vi "chargetest.vi"(0 "stop":bool, 4 "Stop Time(s)":dbl, 5 "Stop Current(A)":dbl, 6 "Stop Capacity(Ah)":dbl, 7 "Stop Voltage(V)":dbl, 8 "Charge\\Discharge Current(A)":dbl, 9 "Charge\\Discharge Voltage(V)":dbl, 10 "Battery Mode":u8(ring) items=["Charge", "Discharge"], 11 "VISA resource name":refnum<visa-resource-name>) -> (1 "Read Voltage(V)":dbl format="%.2g", 2 "Read Current(A)":dbl format="%.2g")   [LabVIEW 2020]
uses:
  <instrlib>/IT-M3400/IT-M3400.lvlib
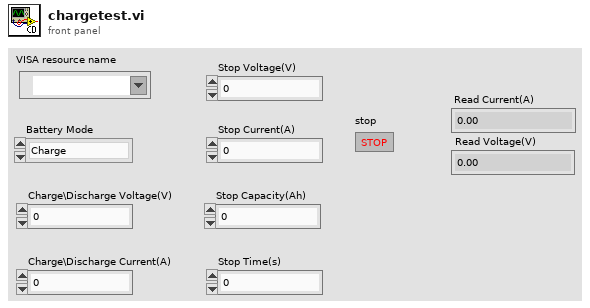
[diagram p1: front panel]
types:
  T1 = cluster{"Baud Rate":u32, "Parity":u16, "Data Bits":u16, "Stop Bits":u16, "Flow Control":u16}
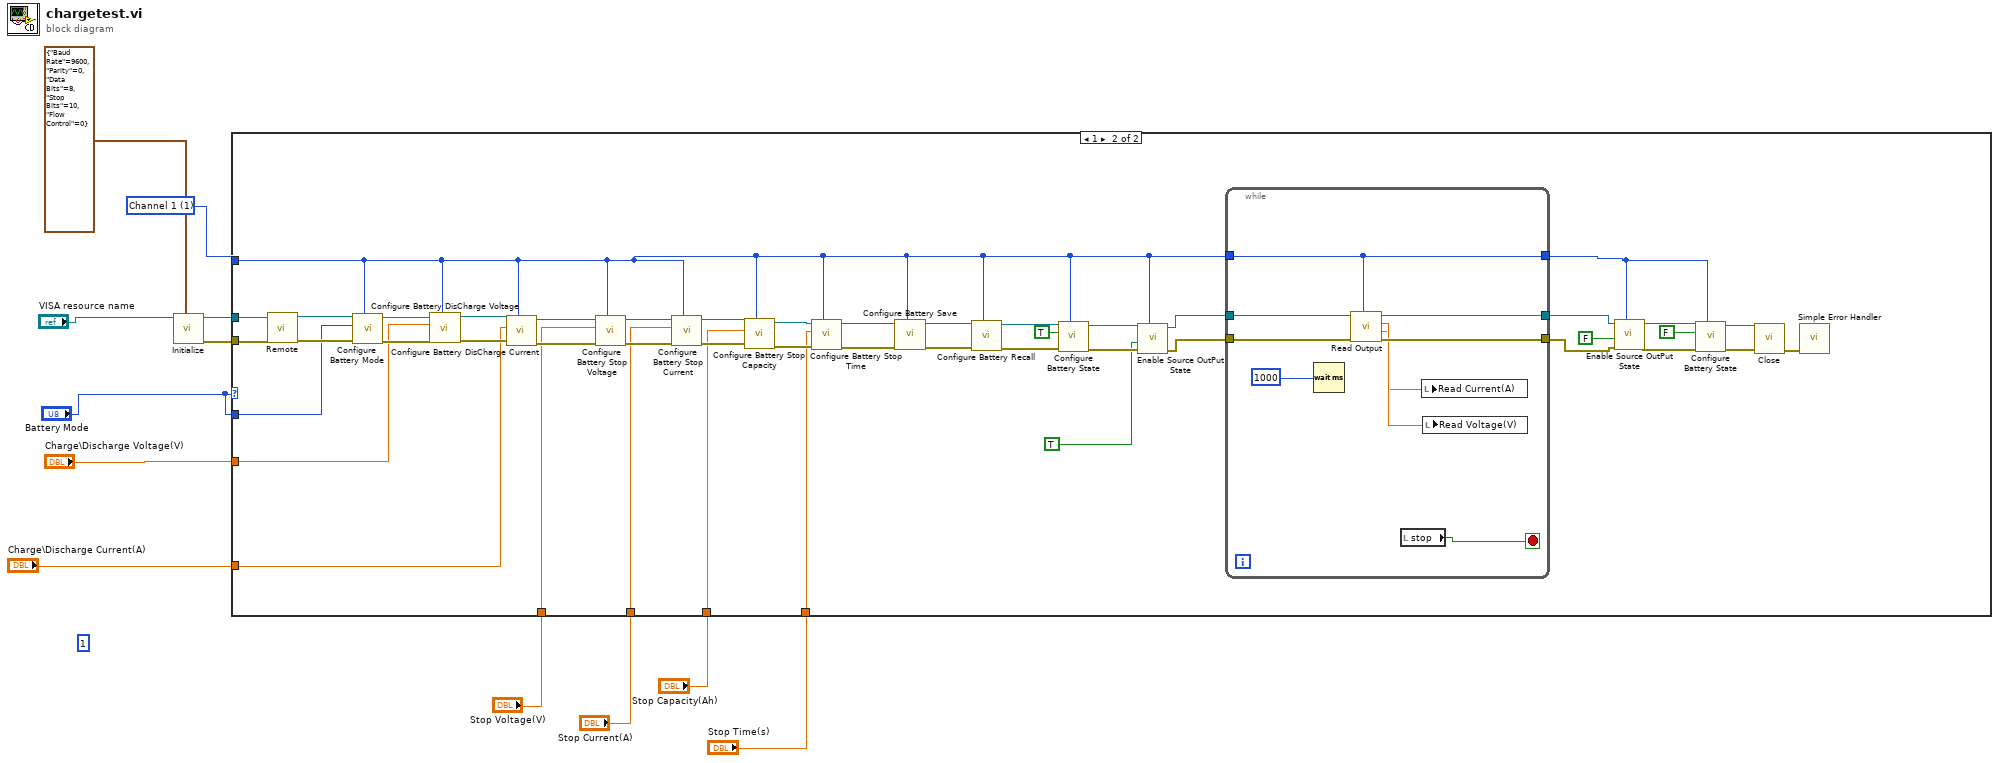
[diagram p0: block diagram]
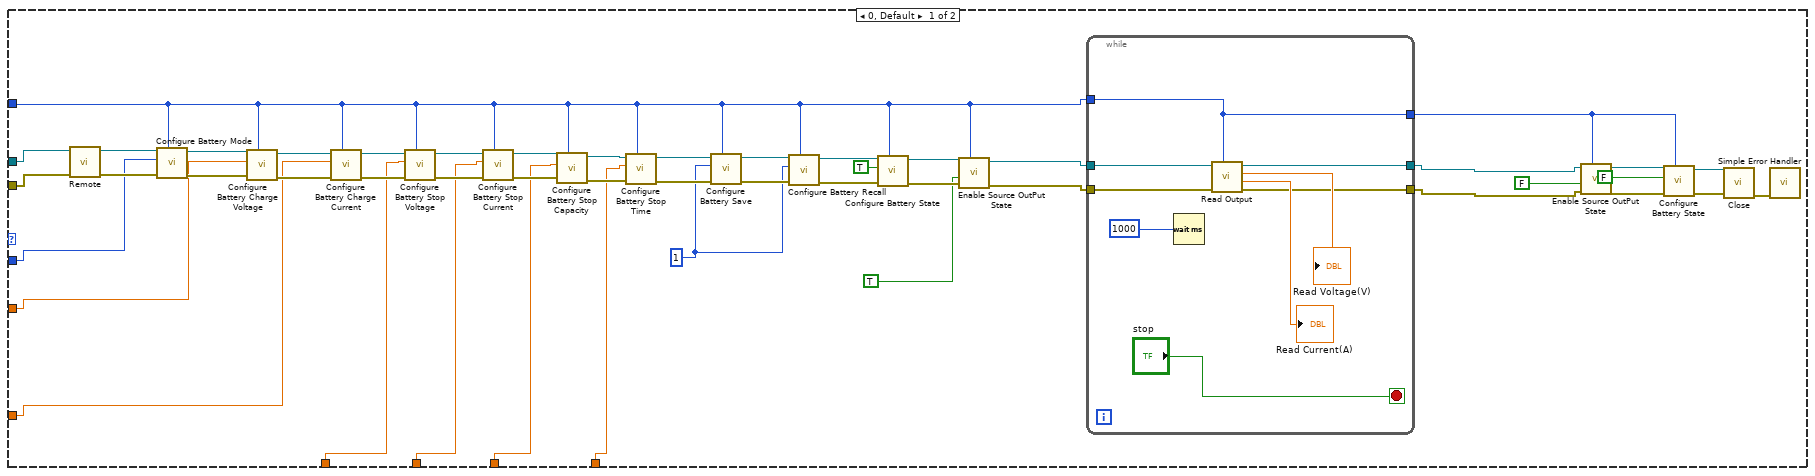
[diagram p2: hidden frame]
diagram:
  w2 = 1 items=["Channel 1"=1, "Channel 2"=2, "Channel 3"=3, "Channel 4"=4, "Channel 5"=5, "Channel 6"=6, "Channel 7"=7, "Channel 8"=8, "Channel 8"=9, "Channel 10"=10, "Channel 11"=11, "Channel 12"=12, "Channel 13"=13, "Channel 14"=14, "Channel 15"=15, "Channel 16"=16] ("Channel")
  (unwired) 1
  n1 = call <instrlib>:"Initialize.vi"("Serial Configuration"=T1 {"Baud Rate"=9600, "Parity"=0, "Data Bits"=8, "Stop Bits"=10, "Flow Control"=0}, "VISA resource name"="VISA resource name") -> ("error out"=w11:errorcluster, "VISA resource name out"=w12:refnum<visa-resource-name>)  [unwired: 8 in]
  n2 = case shown="1" "Battery Mode" {
    tunnel: "Battery Mode" -> [w26 w104]
    tunnel: w12 -> [w28 w103]
    tunnel: w11 -> [w27 w102]
    tunnel: "Charge\\Discharge Voltage(V)" -> [w25 w79]
    tunnel: "Charge\\Discharge Current(A)" -> [w24 w80]
    tunnel: "Stop Voltage(V)" -> [w23 w78]
    tunnel: "Stop Current(A)" -> [w22 w77]
    tunnel: "Stop Capacity(Ah)" -> [w21 w76]
    tunnel: "Stop Time(s)" -> [w20 w75]
    tunnel: w2 -> [w14 w72]
    frame 0, Default {
      w19 = u8 1 ("File")
      n3 = call <instrlib>:"Remote.vi"("error in"=w27, "VISA resource name"=w28) -> ("error out"=w58:errorcluster, "VISA resource name out"=w59:refnum<visa-resource-name>)  [unwired: 8 in]
      n4 = call <instrlib>:"Configure Battery Mode.vi"("Channel"=w14, "error in"=w58, "Battery Mode"=w26, "VISA resource name"=w59) -> ("error out"=w56:errorcluster, "VISA resource name out"=w57:refnum<visa-resource-name>)  [unwired: 6 in]
      n5 = call <instrlib>:"Configure Battery Charge Voltage.vi"("Channel"=w14, "error in"=w56, "Charge Voltage(V)"=w25, "VISA resource name"=w57) -> ("error out"=w54:errorcluster, "VISA resource name out"=w55:refnum<visa-resource-name>)  [unwired: 5 in]
      n6 = call <instrlib>:"Configure Battery Charge Current.vi"("Channel"=w14, "error in"=w54, "Charge Current(A)"=w24, "VISA resource name"=w55) -> ("error out"=w52:errorcluster, "VISA resource name out"=w53:refnum<visa-resource-name>)  [unwired: 6 in]
      n7 = call <instrlib>:"Configure Battery Stop Voltage.vi"("Channel"=w14, "error in"=w52, "Stop Voltage(V)"=w23, "VISA resource name"=w53) -> ("error out"=w50:errorcluster, "VISA resource name out"=w51:refnum<visa-resource-name>)  [unwired: 6 in]
      n8 = call <instrlib>:"Configure Battery Stop Current.vi"("Channel"=w14, "error in"=w50, "Stop Current(A)"=w22, "VISA resource name"=w51) -> ("error out"=w48:errorcluster, "VISA resource name out"=w49:refnum<visa-resource-name>)  [unwired: 6 in]
      n9 = call <instrlib>:"Configure Battery Stop Capacity.vi"("Channel"=w14, "error in"=w48, "Stop Capacity(Ah)"=w21, "VISA resource name"=w49) -> ("error out"=w46:errorcluster, "VISA resource name out"=w47:refnum<visa-resource-name>)  [unwired: 6 in]
      n10 = call <instrlib>:"Configure Battery Stop Time.vi"("Channel"=w14, "error in"=w46, "Stop Time(S)"=w20, "VISA resource name"=w47) -> ("error out"=w44:errorcluster, "VISA resource name out"=w45:refnum<visa-resource-name>)  [unwired: 6 in]
      n11 = call <instrlib>:"Configure Battery Save.vi"("Channel"=w14, "error in"=w44, "File"=w19, "VISA resource name"=w45) -> ("error out"=w42:errorcluster, "VISA resource name out"=w43:refnum<visa-resource-name>)  [unwired: 6 in]
      n12 = call <instrlib>:"Configure Battery Recall.vi"("Channel"=w14, "error in"=w42, "File"=w19, "VISA resource name"=w43) -> ("error out"=w40:errorcluster, "VISA resource name out"=w41:refnum<visa-resource-name>)  [unwired: 6 in]
      n13 = call <instrlib>:"Configure Battery State.vi"("Channel"=w14, "error in"=w40, "State"=TRUE, "VISA resource name"=w41) -> ("error out"=w38:errorcluster, "VISA resource name out"=w39:refnum<visa-resource-name>)  [unwired: 6 in]
      n14 = call <instrlib>:"Enable Source OutPut State.vi"("Channel"=w14, "error in"=w38, "State"=TRUE ("Enable Output|Intput"), "VISA resource name"=w39) -> ("error out"=w17:errorcluster, "VISA resource name out"=w18:refnum<visa-resource-name>)  [unwired: 6 in]
      n15 = while {
        tunnel: w18 -> [w66]
        tunnel: w17 -> [w65]
        tunnel: [w64] -> w16
        tunnel: [w63] -> w15
        tunnel: w14 -> [w60]
        tunnel: [w60] -> w13
        stop <- "stop" stop-if-true
        n16 = Wait (ms)(milliseconds to wait=1000) -> ()  [unwired: 1 out]
        n17 = call <instrlib>:"Read Output.vi"("Channel"=w60, "error in"=w65, "VISA resource name"=w66) -> ("error out"=w63:errorcluster, "Read Current(A)"=→"Read Current(A)":dbl, "Read Voltage(V)"=→"Read Voltage(V)":dbl, "VISA resource name out"=w64:refnum<visa-resource-name>)  [unwired: 5 in]
      }
      n18 = call <instrlib>:"Enable Source OutPut State.vi"("Channel"=w13, "error in"=w15, "State"=FALSE, "VISA resource name"=w16) -> ("error out"=w31:errorcluster, "VISA resource name out"=w34:refnum<visa-resource-name>)  [unwired: 6 in]
      n19 = call <instrlib>:"Configure Battery State.vi"("Channel"=w13, "error in"=w31, "State"=FALSE, "VISA resource name"=w34) -> ("error out"=w32:errorcluster, "VISA resource name out"=w33:refnum<visa-resource-name>)  [unwired: 6 in]
      n20 = call <instrlib>:"Close.vi"("error in"=w32, "VISA resource name"=w33) -> ("error out"=w36:errorcluster)  [unwired: 9 in]
      n21 = call <vilib>:"Simple Error Handler.vi"("error in (no error)"=w36) -> ()  [unwired: 4 in, 5 out]
    }
    frame 1 {
      n22 = call <instrlib>:"Remote.vi"("error in"=w102, "VISA resource name"=w103) -> ("error out"=w113:errorcluster, "VISA resource name out"=w114:refnum<visa-resource-name>)  [unwired: 8 in]
      n23 = call <instrlib>:"Configure Battery Mode.vi"("Channel"=w72, "error in"=w113, "Battery Mode"=w104, "VISA resource name"=w114) -> ("error out"=w85:errorcluster, "VISA resource name out"=w86:refnum<visa-resource-name>)  [unwired: 6 in]
      n24 = call <instrlib>:"Configure Battery DisCharge Voltage.vi"("Channel"=w72, "error in"=w85, "Discharge Voltage(V)"=w79, "VISA resource name"=w86) -> ("error out"=w83:errorcluster, "VISA resource name out"=w84:refnum<visa-resource-name>)  [unwired: 6 in]
      n25 = call <instrlib>:"Configure Battery DisCharge Current.vi"("Channel"=w72, "error in"=w83, "Discharge Current(A)"=w80, "VISA resource name"=w84) -> ("error out"=w81:errorcluster, "VISA resource name out"=w82:refnum<visa-resource-name>)  [unwired: 6 in]
      n26 = call <instrlib>:"Configure Battery Stop Voltage.vi"("Channel"=w72, "error in"=w81, "Stop Voltage(V)"=w78, "VISA resource name"=w82) -> ("error out"=w111:errorcluster, "VISA resource name out"=w112:refnum<visa-resource-name>)  [unwired: 6 in]
      n27 = call <instrlib>:"Configure Battery Stop Current.vi"("Channel"=w72, "error in"=w111, "Stop Current(A)"=w77, "VISA resource name"=w112) -> ("error out"=w109:errorcluster, "VISA resource name out"=w110:refnum<visa-resource-name>)  [unwired: 6 in]
      n28 = call <instrlib>:"Configure Battery Stop Capacity.vi"("Channel"=w72, "error in"=w109, "Stop Capacity(Ah)"=w76, "VISA resource name"=w110) -> ("error out"=w107:errorcluster, "VISA resource name out"=w108:refnum<visa-resource-name>)  [unwired: 6 in]
      n29 = call <instrlib>:"Configure Battery Stop Time.vi"("Channel"=w72, "error in"=w107, "Stop Time(S)"=w75, "VISA resource name"=w108) -> ("error out"=w105:errorcluster, "VISA resource name out"=w106:refnum<visa-resource-name>)  [unwired: 6 in]
      n30 = call <instrlib>:"Configure Battery Save.vi"("Channel"=w72, "error in"=w105, "VISA resource name"=w106) -> ("error out"=w100:errorcluster, "VISA resource name out"=w101:refnum<visa-resource-name>)  [unwired: 7 in]
      n31 = call <instrlib>:"Configure Battery Recall.vi"("Channel"=w72, "error in"=w100, "VISA resource name"=w101) -> ("error out"=w98:errorcluster, "VISA resource name out"=w99:refnum<visa-resource-name>)  [unwired: 7 in]
      n32 = call <instrlib>:"Configure Battery State.vi"("Channel"=w72, "error in"=w98, "State"=TRUE, "VISA resource name"=w99) -> ("error out"=w96:errorcluster, "VISA resource name out"=w97:refnum<visa-resource-name>)  [unwired: 6 in]
      n33 = call <instrlib>:"Enable Source OutPut State.vi"("Channel"=w72, "error in"=w96, "State"=TRUE ("Enable Output|Intput"), "VISA resource name"=w97) -> ("error out"=w73:errorcluster, "VISA resource name out"=w74:refnum<visa-resource-name>)  [unwired: 6 in]
      n34 = while {
        tunnel: [w123] -> w71
        tunnel: [w122] -> w70
        tunnel: w74 -> [w120]
        tunnel: w73 -> [w119]
        tunnel: w72 -> [w118]
        tunnel: [w118] -> w69
        stop <- w115 stop-if-true
        n35 = Wait (ms)(milliseconds to wait=1000) -> ()  [unwired: 1 out]
        n36 = call <instrlib>:"Read Output.vi"("Channel"=w118, "error in"=w119, "VISA resource name"=w120) -> ("error out"=w122:errorcluster, "Read Current(A)"=w116:dbl, "Read Voltage(V)"=w117:dbl, "VISA resource name out"=w123:refnum<visa-resource-name>)  [unwired: 5 in]
        n37 = local read "stop"() -> (w115:bool)
        n38 = local write "Read Current(A)"(w116) -> ()
        n39 = local write "Read Voltage(V)"(w117) -> ()
      }
      n40 = call <instrlib>:"Enable Source OutPut State.vi"("Channel"=w69, "error in"=w70, "State"=FALSE, "VISA resource name"=w71) -> ("error out"=w89:errorcluster, "VISA resource name out"=w92:refnum<visa-resource-name>)  [unwired: 6 in]
      n41 = call <instrlib>:"Configure Battery State.vi"("Channel"=w69, "error in"=w89, "State"=FALSE, "VISA resource name"=w92) -> ("error out"=w90:errorcluster, "VISA resource name out"=w91:refnum<visa-resource-name>)  [unwired: 6 in]
      n42 = call <instrlib>:"Close.vi"("error in"=w90, "VISA resource name"=w91) -> ("error out"=w94:errorcluster)  [unwired: 9 in]
      n43 = call <vilib>:"Simple Error Handler.vi"("error in (no error)"=w94) -> ()  [unwired: 4 in, 5 out]
    }
  }
